vi "FGV FID CH4 Kalibrieren.vi"(10 "Aktionen FID kalibrieren":T1, 11 "Sprachliste":string[][](array[string])) -> (1 "Zustand PMA":string, 2 "Aktionen FID kalibrieren":T1)   [LabVIEW 2020, in "Auto Kalibrieren.lvlib"]
uses:
  Auto Kalibrieren.lvlib
  Aktionen FID kalibrieren.ctl
  Analysator Definition/FGV Analysator Definition Aktionen.ctl
  Aktion FGV CalZustand.ctl
  Seiten/EL3000/FID/Aktion FGV Messwerte_F.ctl
  Aktionen FGV Zustand Kalibrierung.ctl
  Aktionen FGV AutoKAL Daten.ctl
  Seiten/EL3000/Allgemeine VI/FGV Uras26 Aktion.ctl
  Seiten/EL3000/FID/FID Kalibrierung/FID Kalibrieren.ctl
  Seiten/EL3000/Allgemeine VI/Allgemeine VI.lvlib
  Seiten/EL3000/FID/FID.lvlib
  Seiten/EL3000/FID/FID Kalibrierung/FID Kalibrierung.lvlib
  Analysator Definition/Analysator Definition.lvlib
  Seiten/CalGas Aufschaltung/CalGas Aufschaltung.lvlib
  Sprachverwaltung/Sprachverwaltung.lvlib
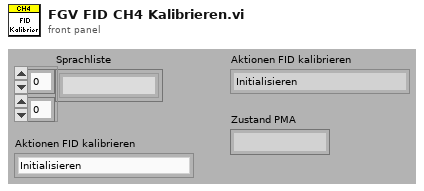
[diagram p1: front panel]
types:
  T1 = typedef "Auto Kalibrieren.lvlib/Aktionen FID kalibrieren.ctl" = enum16{"Initialisieren", "Warten auf FTIR", "Anstehende Störung", "0-Gas Aufschalten", "Nullpunkt Anfordern", "Nullpunkt", "Warten auf andere Messgeräte", "Messgas Aufschalten", "Endpunkt Anfordern", "Endpunkt", "Endpunkt kopieren", "Fertig", "Speichern"}
  T2 = typedef "Analysator Definition.lvlib/FGV Analysator Definition Aktionen.ctl" = enum16{"lesen", "MB setzen", "MB KAL setzen", "laden"}
  T3 = typedef "ABB-EL3000.lvlib/FID.lvlib/Aktion FGV Messwerte_F.ctl" = enum16{"lesen", "Messwerte", "Messbereich", "Status", "Diagnose Werte"}
  T4 = typedef "Auto Kalibrieren.lvlib/Aktion FGV CalZustand.ctl" = enum16{"lesen", "Cal FTIR", "Cal FID CH4", "Cal PMA", "init", "Cal FID THC", "THC CG Eingang"}
  T5 = typedef "Auto Kalibrieren.lvlib/Aktionen FGV Zustand Kalibrierung.ctl" = enum16{"lesen", "LÖSCHEN", "Hintergrund fertig", "Nullpunkt NDIR CO lo", "Endpunkt NDIR CO lo", "Nullpunkt NDIR CO hi", "Endpunkt NDIR CO hi", "Nullpunkt NDIR CO2 lo", "Endpunkt NDIR CO2 lo", "Nullpunkt FID CH4", "Endpunkt FID CH4", "Nullpunkt FID THC", "Endpunkt FID THC", "Nullpunkt PMA", "Endpunkt PMA", "Fehler FT-IR", "Fehler NDIR lo", "Fehler FID CH4", "Fehler FID THC", "Fehler PMA", "TIMEOUT"}
  T6 = typedef "Auto Kalibrieren.lvlib/Aktionen FGV AutoKAL Daten.ctl" = enum16{"lesen", "laden", "speichern", "Aufschaltzeit"}
  T7 = typedef "ABB-EL3000.lvlib/FID.lvlib/FID Kalibrierung.lvlib/FID Kalibrieren.ctl" = enum16{"CH4 Nullpunkt", "THC Nullpunkt", "NMHC Nullpunkt", "CH4 Endpunkt", "THC Endpunkt", "NMHC Endpunkt"}
  T8 = typedef "ABB-EL3000.lvlib/Allgemeine VI.lvlib/FGV Uras26 Aktion.ctl" = enum16{"lesen", "CAL-Daten laden", "Messen", "Kalibrieren vorbereiten", "Kalibrieren", "CAL-Daten speichern", "Toleranz schreiben", "CAL-Daten kopieren"}
  T9 = typedef "Analysator Definition.lvlib/Betriebsdaten Komponente.ctl" = cluster{"Namen":string[], "MB Namen":string[], "Einheit":string, "MB Aktuell":u16, "MB Endwert":u16, "CalGase":u16[], "MB für KAL":u16[], "CG für KAL":u16[]}
  T10 = cluster{"Ausfall":bool, "Funktionskontrolle":bool, "Wartungsbedarf":bool}
  T11 = typedef "Auto Kalibrieren.lvlib/Auschaltzeiten Null Endpunktgase.ctl" = cluster{"CO lo 0":sgl, "CO lo E":sgl, "CO hi 0":sgl, "CO hi E":sgl, "CO2 lo 0":sgl, "CO2 lo E":sgl, "CH4 0":sgl, "CH4 E":sgl, "THC 0":sgl, "THC E":sgl, "O2 0":sgl, "O2 E":sgl}
  T12 = typedef "Auto Kalibrieren.lvlib/Zustand Messgeraete Kalibrierung.ctl" = cluster{"Hintergrund FT-IR":bool, "Nullpunkt NDIR CO lo":bool, "Endpunkt NDIR CO lo":bool, "Nullpunkt NDIR CO hi":bool, "Endpunkt NDIR CO hi":bool, "Nullpunkt NDIR CO2 lo":bool, "Endpunkt NDIR CO2 lo":bool, "Nullpunkt FID CH4":bool, "Endpunkt FID CH4":bool, "Nullpunkt FID THC":bool, "Endpunkt FID THC":bool, "Nullpunkt PMA":bool, "Endpunkt PMA":bool, "Fehler FT-IR":bool, "Fehler NDIR lo":bool, "Fehler FID CH4":bool, "Fehler FID THC":bool, "Fehler PMA":bool}
  T13 = typedef "Zahlen-Ausgabefeld.ctl" = sgl
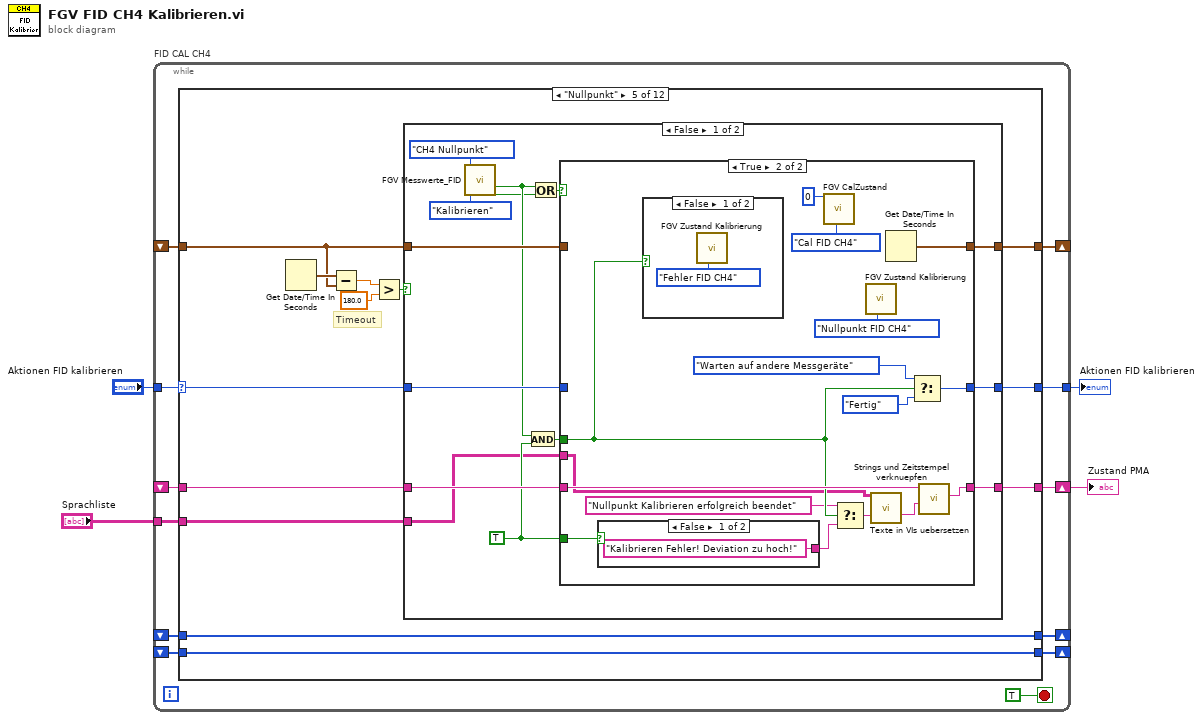
[diagram p0: block diagram]
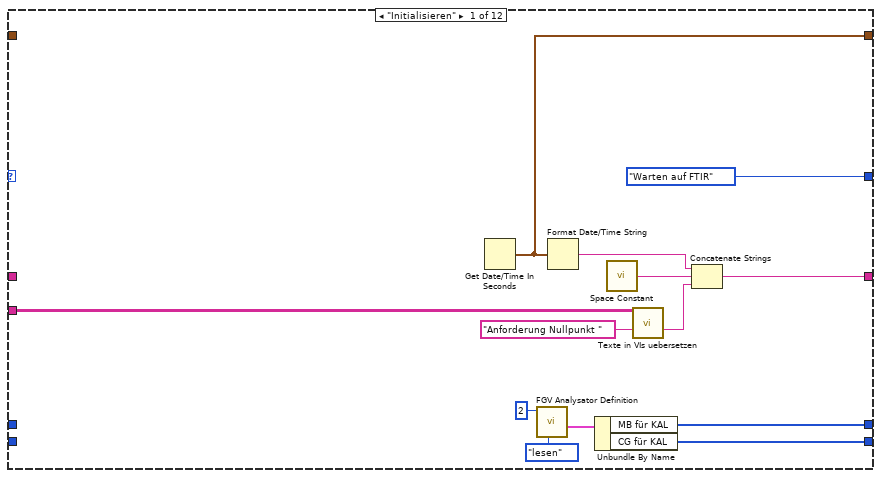
[diagram p2: hidden frame]
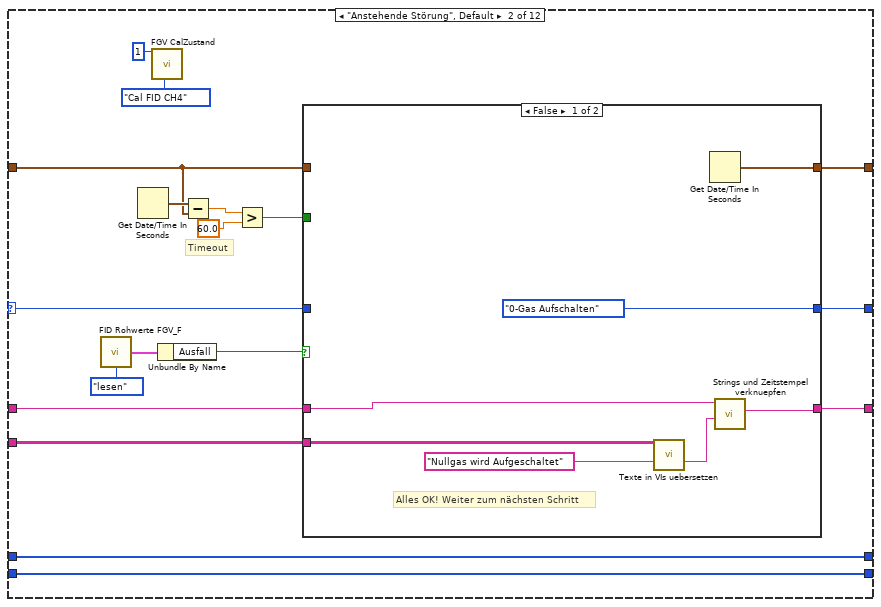
[diagram p3: hidden frame]
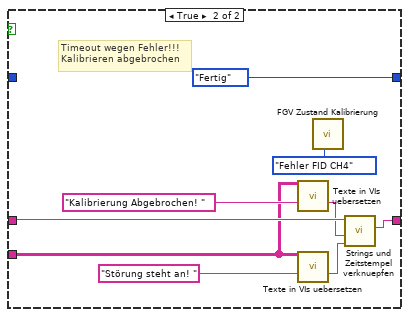
[diagram p5: hidden frame]
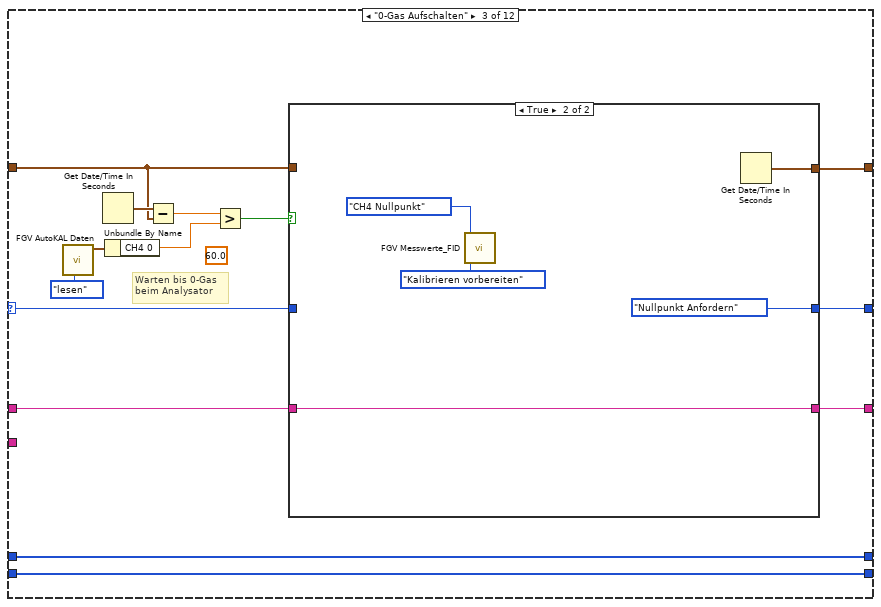
[diagram p6: hidden frame]
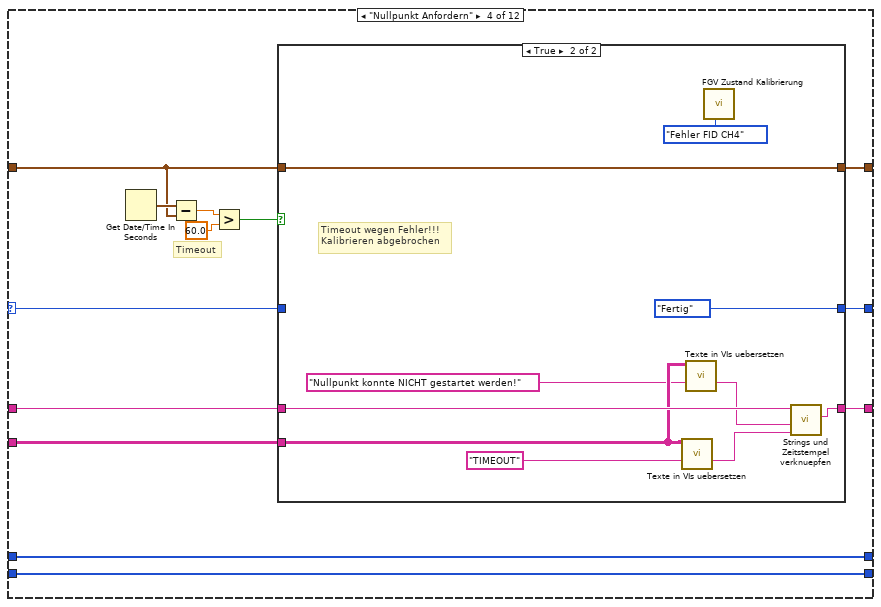
[diagram p8: hidden frame]
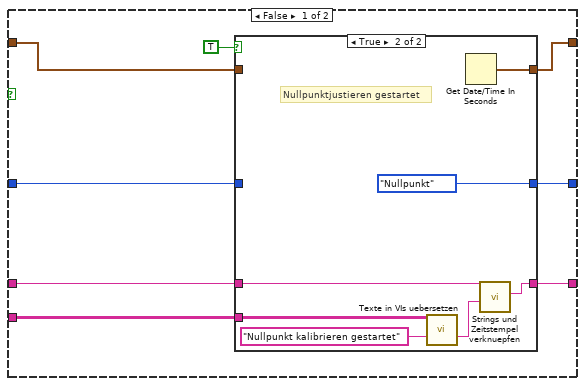
[diagram p9: hidden frame]
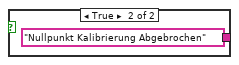
[diagram p12: hidden frame]
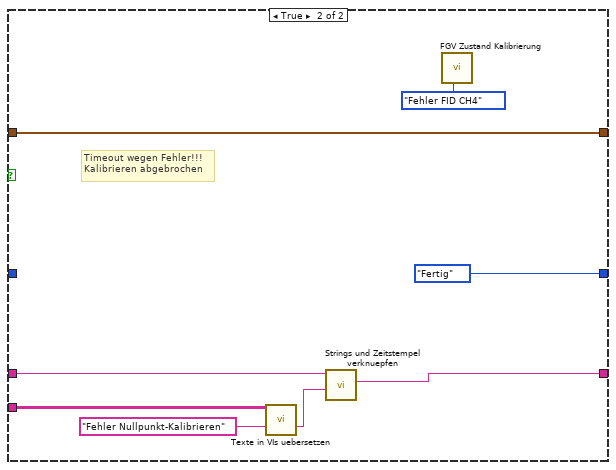
[diagram p14: hidden frame]
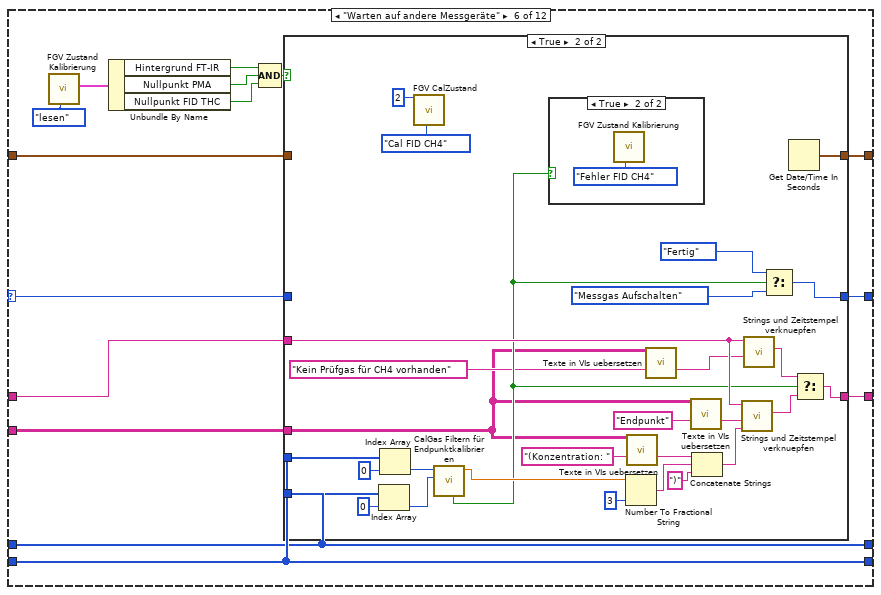
[diagram p15: hidden frame]
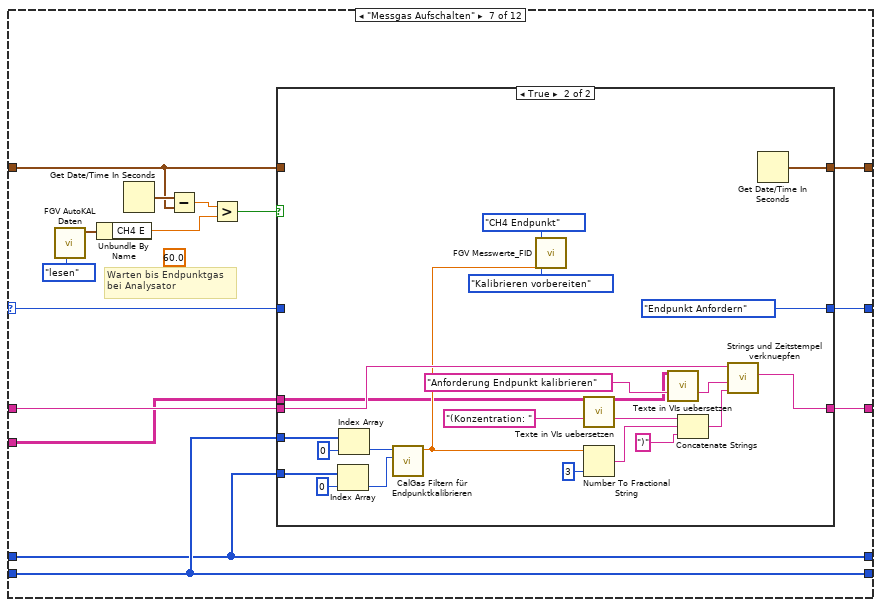
[diagram p18: hidden frame]
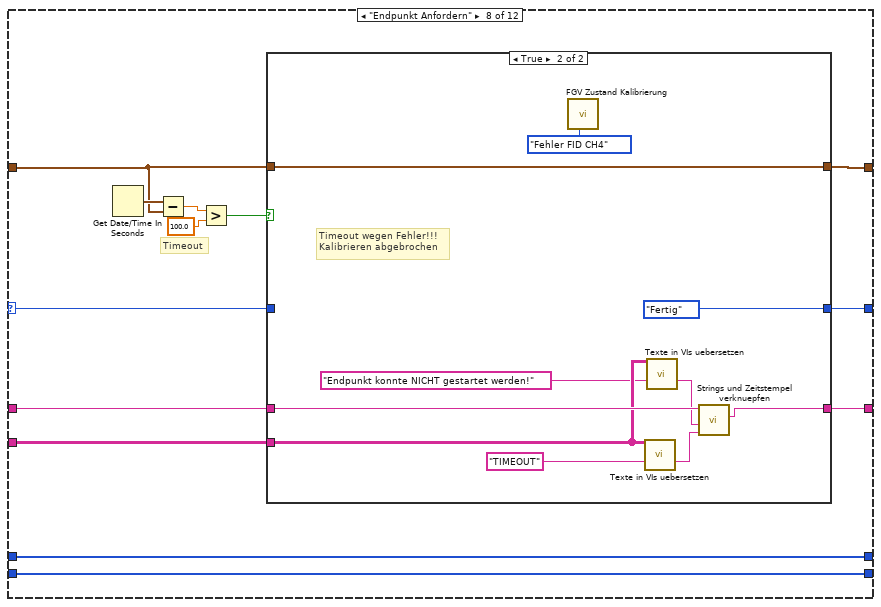
[diagram p20: hidden frame]
diagram:
  n1 = while "FID CAL CH4" {
    shift-right: [w12] -> w4
    shift-left: _ -> [w14]
    shift-right: [w13] -> _
    shift-left: _ -> [w15]
    tunnel: "Aktionen FID kalibrieren" -> [w16]
    tunnel: [w11] -> w2
    shift-right: [w8] -> _
    shift-left: _ -> [w6]
    shift-right: [w9] -> _
    shift-left: _ -> [w7]
    tunnel: "Sprachliste" -> [w5]
    stop <- TRUE stop-if-true
    n2 = case shown="\"Nullpunkt\"" w16 {
      selector: w16 -> [_ w40 w81 w98 w139 w202 w250 w285 w330 w383 _ w404]
      tunnel: w15 -> [_ w38 w83 w103 w141 w203 w253 w290 w332 w384 _ w405]
      tunnel: w14 -> [_ w43 w79 w100 w143 w205 w248 w287 w331 w382 w397 w409]
      tunnel: [w27 w44 w82 w102 w140 w206 w252 w289 w329 w384 w398 w405] -> w13
      tunnel: [w26 w42 w78 w99 w142 w204 w247 w286 w327 w382 w397 w409] -> w12
      tunnel: [Aktionen_FID_kalibrieren."Warten auf FTIR" ("Aktionen FID kalibrieren") w39 w80 w101 w144 w207 w249 w288 w328 w383 Aktionen_FID_kalibrieren."Fertig" ("Aktionen FID kalibrieren") w408] -> w11
      tunnel: [w21 w32 w74 w97 w138 w195 w242 w284 w325 w381 w394 w401] -> w9
      tunnel: [w20 w31 w73 w96 w137 w196 w243 w283 w324 w380 w393 w400] -> w8
      tunnel: w7 -> [_ w32 w74 w97 w138 w195 w242 w284 w325 w381 w394 w401]
      tunnel: w6 -> [_ w31 w73 w96 w137 w196 w243 w283 w324 w380 w393 w400]
      tunnel: w5 -> [w17 w30 _ w95 w136 w193 w241 w282 w323 _ _ _]
      frame "Initialisieren" {
        n3 = Get Date/Time In Seconds() -> (seconds since 1Jan1904=w27:timestamp)
        n4 = call "FGV Analysator Definition.vi"("Aktionen"=FGV_Analysator_Definition_Aktionen."lesen", "Komponente"=2) -> ("Betriebsdaten Komponente"=w23:T9)  [unwired: 5 in, 4 out]
        n5 = Format Date/Time String(seconds (now)=w27) -> (date/time string=w29:string)  [unwired: 2 in]
        n6 = Unbundle By Name(w23) -> ("MB für KAL"=w21:u16[], "CG für KAL"=w20:u16[])
        n7 = call <vilib>:"Space Constant.vi"() -> ("String"=w28:string)
        n8 = call "Texte in VIs uebersetzen.vi"("Sprachliste"=w17, "String zum Übersetzen"="Anforderung Nullpunkt " ("String")) -> ("String zum Übersetzen"=w18:string)  [unwired: 9 in, 4 out]
        n9 = Concatenate Strings(w29, w28, w18) -> (w26:string)
      }
      frame "Anstehende Störung", Default {
        # "Timeout"
        n10 = call "FID Rohwerte FGV_F.vi"("Aktion"=Aktion_FGV_Messwerte_F."lesen") -> ("Status"=w36:T10)  [unwired: 11 in, 3 out]
        n11 = Get Date/Time In Seconds() -> (seconds since 1Jan1904=w47:timestamp)
        n12 = call "FGV CalZustand.vi"("CAL Zustand"=u16 1 ("CAL Zustand FTIR"), "Aktion"=Aktion_FGV_CalZustand."Cal FID CH4") -> ()  [unwired: 13 in, 5 out]
        n13 = Unbundle By Name(w36) -> ("Ausfall"=w37:bool)
        n14 = Subtract(x=w47, y=w38) -> (x-y=w46:dbl)
        n15 = Greater?(x=w46, y=60.0) -> (0:w41:bool)
        n16 = case shown="False" w37 {
          tunnel: [w54 w58] -> w44
          tunnel: w43 -> [w53 w57]
          tunnel: [w52 w56] -> w42
          tunnel: w41 -> [_ w61]
          tunnel: w40 -> [_ w60]
          tunnel: [Aktionen_FID_kalibrieren."0-Gas Aufschalten" ("Aktionen FID kalibrieren") w59] -> w39
          tunnel: w38 -> [_ w58]
          tunnel: w30 -> [w48 w55]
          frame False {
            # "Alles OK! Weiter zum nächsten Schritt"
            n17 = call "Texte in VIs uebersetzen.vi"("Sprachliste"=w48, "String zum Übersetzen"="Nullgas wird Aufgeschaltet" ("String 1 hinzufügen")) -> ("String zum Übersetzen"=w49:string)  [unwired: 9 in, 4 out]
            n18 = Get Date/Time In Seconds() -> (seconds since 1Jan1904=w54:timestamp)
            n19 = call "Strings und Zeitstempel verknuepfen.vi"("String 1 hinzufügen"=w49, "Eingagns String"=w53) -> ("Verknüpfter String"=w52:string)  [unwired: 9 in]
          }
          frame True {
            n20 = case shown="False" w61 {
              tunnel: w60 -> [w63 _]
              tunnel: [w63 Aktionen_FID_kalibrieren."Fertig" ("Aktionen FID kalibrieren")] -> w59
              tunnel: w57 -> [w62 w72]
              tunnel: [w62 w71] -> w56
              tunnel: w55 -> [_ w65]
              frame False {
                # "Fehler steht an!!!!"
              }
              frame True {
                # "Timeout wegen Fehler!!! \nKalibrieren abgebrochen"
                n21 = call "Texte in VIs uebersetzen.vi"("Sprachliste"=w65, "String zum Übersetzen"="Kalibrierung Abgebrochen! " ("String")) -> ("String zum Übersetzen"=w67:string)  [unwired: 9 in, 4 out]
                n22 = call "Texte in VIs uebersetzen.vi"("Sprachliste"=w65, "String zum Übersetzen"="Störung steht an! " ("String")) -> ("String zum Übersetzen"=w66:string)  [unwired: 9 in, 4 out]
                n23 = call "FGV Zustand Kalibrierung.vi"("Aktionen"=Aktionen_FGV_Zustand_Kalibrierung."Fehler FID CH4" ("Enum")) -> ()  [unwired: 9 in, 2 out]
                n24 = call "Strings und Zeitstempel verknuepfen.vi"("String 2 hinzufügen"=w66, "String 1 hinzufügen"=w67, "Eingagns String"=w72) -> ("Verknüpfter String"=w71:string)  [unwired: 8 in]
              }
            }
          }
        }
      }
      frame "0-Gas Aufschalten" {
        (unwired) 60.0 ("y")
        # "Warten bis 0-Gas \nbeim Analysator"
        n25 = call "FGV AutoKAL Daten.vi"("Aktionen"=Aktionen_FGV_AutoKAL_Daten."lesen") -> ("Aufschaltzeiten"=w76:T11)  [unwired: 10 in]
        n26 = Get Date/Time In Seconds() -> (seconds since 1Jan1904=w86:timestamp)
        n27 = Unbundle By Name(w76) -> ("CH4 0"=w75:sgl)
        n28 = Subtract(x=w86, y=w83) -> (x-y=w85:dbl)
        n29 = Greater?(x=w85, y=w75) -> (0:w84:bool)
        n30 = case shown="True" w84 {
          tunnel: w83 -> [w89 _]
          tunnel: [w89 w94] -> w82
          tunnel: w81 -> [w88 _]
          tunnel: [w88 Aktionen_FID_kalibrieren."Nullpunkt Anfordern" ("Aktionen FID kalibrieren")] -> w80
          tunnel: w79 -> [w87 w93]
          tunnel: [w87 w93] -> w78
          frame False {
          }
          frame True {
            n31 = call "FGV Messwerte_FID.vi"("Kalibrieren"=FID_Kalibrieren."CH4 Nullpunkt", "Aktion"=FGV_Uras26_Aktion."Kalibrieren vorbereiten") -> ()  [unwired: 18 in, 8 out]
            n32 = Get Date/Time In Seconds() -> (seconds since 1Jan1904=w94:timestamp)
          }
        }
      }
      frame "Nullpunkt Anfordern" {
        # "Timeout"
        n33 = Get Date/Time In Seconds() -> (seconds since 1Jan1904=w107:timestamp)
        n34 = Subtract(x=w107, y=w103) -> (x-y=w106:dbl)
        n35 = Greater?(x=w106, y=60.0) -> (0:w104:bool)
        n36 = case shown="True" w104 {
          tunnel: w103 -> [w111 w135]
          tunnel: [w110 w135] -> w102
          tunnel: [w113 Aktionen_FID_kalibrieren."Fertig" ("Aktionen FID kalibrieren")] -> w101
          tunnel: w100 -> [w115 w134]
          tunnel: [w114 w133] -> w99
          tunnel: w98 -> [w112 _]
          tunnel: w95 -> [w108 w127]
          frame False {
            n37 = case shown="True" TRUE {
              tunnel: w115 -> [w116 w125]
              tunnel: [w116 w124] -> w114
              tunnel: [w118 Aktionen_FID_kalibrieren."Nullpunkt" ("Aktionen FID kalibrieren")] -> w113
              tunnel: w112 -> [w118 _]
              tunnel: w111 -> [w117 _]
              tunnel: [w117 w123] -> w110
              tunnel: w108 -> [_ w119]
              frame False {
              }
              frame True {
                # "Nullpunktjustieren gestartet"
                n38 = call "Texte in VIs uebersetzen.vi"("Sprachliste"=w119, "String zum Übersetzen"="Nullpunkt kalibrieren gestartet" ("String 1 hinzufügen")) -> ("String zum Übersetzen"=w120:string)  [unwired: 9 in, 4 out]
                n39 = Get Date/Time In Seconds() -> (seconds since 1Jan1904=w123:timestamp)
                n40 = call "Strings und Zeitstempel verknuepfen.vi"("String 1 hinzufügen"=w120, "Eingagns String"=w125) -> ("Verknüpfter String"=w124:string)  [unwired: 9 in]
              }
            }
          }
          frame True {
            # "Timeout wegen Fehler!!! \nKalibrieren abgebrochen"
            n41 = call "Texte in VIs uebersetzen.vi"("Sprachliste"=w127, "String zum Übersetzen"="TIMEOUT" ("String")) -> ("String zum Übersetzen"=w128:string)  [unwired: 9 in, 4 out]
            n42 = call "Texte in VIs uebersetzen.vi"("Sprachliste"=w127, "String zum Übersetzen"="Nullpunkt konnte NICHT gestartet werden!" ("String")) -> ("String zum Übersetzen"=w130:string)  [unwired: 9 in, 4 out]
            n43 = call "FGV Zustand Kalibrierung.vi"("Aktionen"=Aktionen_FGV_Zustand_Kalibrierung."Fehler FID CH4" ("Enum")) -> ()  [unwired: 9 in, 2 out]
            n44 = call "Strings und Zeitstempel verknuepfen.vi"("String 2 hinzufügen"=w128, "String 1 hinzufügen"=w130, "Eingagns String"=w134) -> ("Verknüpfter String"=w133:string)  [unwired: 8 in]
          }
        }
      }
      frame "Nullpunkt" {
        # "Timeout"
        n45 = Get Date/Time In Seconds() -> (seconds since 1Jan1904=w148:timestamp)
        n46 = Subtract(x=w148, y=w141) -> (x-y=w147:dbl)
        n47 = Greater?(x=w147, y=180.0) -> (0:w145:bool)
        n48 = case shown="False" w145 {
          tunnel: [w159 Aktionen_FID_kalibrieren."Fertig" ("Aktionen FID kalibrieren")] -> w144
          tunnel: w143 -> [w158 w192]
          tunnel: [w157 w191] -> w142
          tunnel: w141 -> [w162 w190]
          tunnel: [w161 w190] -> w140
          tunnel: w139 -> [w160 _]
          tunnel: w136 -> [w149 w186]
          frame False {
            w154 = TRUE
            n49 = call "FGV Messwerte_FID.vi"("Kalibrieren"=FID_Kalibrieren."CH4 Nullpunkt", "Aktion"=FGV_Uras26_Aktion."Kalibrieren") -> ("Kalibrieren erfolgreich"=w151:bool, "CAL TimeOut"=w150:bool)  [unwired: 18 in, 6 out]
            n50 = And(x=w151, y=w154) -> (x .and. y?=w155:bool)
            n51 = Or(x=w151, y=w150) -> (x .or. y?=w156:bool)
            n52 = case shown="True" w156 {
              tunnel: w162 -> [w165 _]
              tunnel: [w165 w177] -> w161
              tunnel: w160 -> [w164 _]
              tunnel: [w164 w178] -> w159
              tunnel: w158 -> [w163 w181]
              tunnel: [w163 w180] -> w157
              tunnel: w155 -> [_ w175]
              tunnel: w154 -> [_ w174]
              tunnel: w149 -> [_ w167]
              frame False {
              }
              frame True {
                n53 = case shown="False" w174 {
                  tunnel: ["Kalibrieren Fehler! Deviation zu hoch!" ("String 1 hinzufügen") "Nullpunkt Kalibrierung Abgebrochen" ("String 1 hinzufügen")] -> w179
                  frame False {
                  }
                  frame True {
                  }
                }
                n54 = case shown="False" w175 {
                  frame False {
                    n55 = call "FGV Zustand Kalibrierung.vi"("Aktionen"=Aktionen_FGV_Zustand_Kalibrierung."Fehler FID CH4" ("Enum")) -> ()  [unwired: 9 in, 2 out]
                  }
                  frame True {
                  }
                }
                n56 = call "FGV CalZustand.vi"("CAL Zustand"=u16 0 ("CAL Zustand FTIR"), "Aktion"=Aktion_FGV_CalZustand."Cal FID CH4") -> ()  [unwired: 13 in, 5 out]
                n57 = Select(t="Nullpunkt Kalibrieren erfolgreich beendet" ("String 1 hinzufügen"), s=w175, f=w179) -> (s? t:f=w169:string)
                n58 = call "FGV Zustand Kalibrierung.vi"("Aktionen"=Aktionen_FGV_Zustand_Kalibrierung."Nullpunkt FID CH4" ("Enum")) -> ()  [unwired: 9 in, 2 out]
                n59 = call "Texte in VIs uebersetzen.vi"("Sprachliste"=w167, "String zum Übersetzen"=w169) -> ("String zum Übersetzen"=w168:string)  [unwired: 9 in, 4 out]
                n60 = Get Date/Time In Seconds() -> (seconds since 1Jan1904=w177:timestamp)
                n61 = Select(t=Aktionen_FID_kalibrieren."Warten auf andere Messgeräte" ("Aktionen FID kalibrieren"), s=w175, f=Aktionen_FID_kalibrieren."Fertig" ("Aktionen FID kalibrieren")) -> (s? t:f=w178:T1)
                n62 = call "Strings und Zeitstempel verknuepfen.vi"("String 1 hinzufügen"=w168, "Eingagns String"=w181) -> ("Verknüpfter String"=w180:string)  [unwired: 9 in]
              }
            }
          }
          frame True {
            # "Timeout wegen Fehler!!! \nKalibrieren abgebrochen"
            n63 = call "Texte in VIs uebersetzen.vi"("Sprachliste"=w186, "String zum Übersetzen"="Fehler Nullpunkt-Kalibrieren" ("String 1 hinzufügen")) -> ("String zum Übersetzen"=w187:string)  [unwired: 9 in, 4 out]
            n64 = call "Strings und Zeitstempel verknuepfen.vi"("String 1 hinzufügen"=w187, "Eingagns String"=w192) -> ("Verknüpfter String"=w191:string)  [unwired: 9 in]
            n65 = call "FGV Zustand Kalibrierung.vi"("Aktionen"=Aktionen_FGV_Zustand_Kalibrierung."Fehler FID CH4" ("Enum")) -> ()  [unwired: 9 in, 2 out]
          }
        }
      }
      frame "Warten auf andere Messgeräte" {
        n66 = call "FGV Zustand Kalibrierung.vi"("Aktionen"=Aktionen_FGV_Zustand_Kalibrierung."lesen" ("Enum")) -> ("Zustand Kalibrierung"=w200:T12)  [unwired: 9 in, 1 out]
        n67 = Unbundle By Name(w200) -> ("Hintergrund FT-IR"=w199:bool, "Nullpunkt PMA"=w197:bool, "Nullpunkt FID THC"=w194:bool)
        n68 = Compound Arithmetic op=AND(w199, w197, w194) -> (w198:bool)
        n69 = case shown="True" w198 {
          tunnel: [w209 w234] -> w207
          tunnel: [w210 w239] -> w206
          tunnel: w205 -> [w208 w236]
          tunnel: [w208 w235] -> w204
          tunnel: w203 -> [w210 _]
          tunnel: w202 -> [w209 _]
          tunnel: w196 -> [_ w219]
          tunnel: w195 -> [_ w218]
          tunnel: w193 -> [_ w211]
          frame False {
          }
          frame True {
            n70 = Index Array(array=w218, index=0 ("Index")) -> (element=w222:u16)
            n71 = Index Array(array=w219, index=0 ("Index")) -> (element=w223:u16)
            n72 = call "FGV CalZustand.vi"("CAL Zustand"=u16 2 ("CAL Zustand FTIR"), "Aktion"=Aktion_FGV_CalZustand."Cal FID CH4") -> ()  [unwired: 13 in, 5 out]
            n73 = call "CalGas Filtern für Endpunktkalibrieren.vi"("Messbereich"=w222, "CalGas"=w223) -> ("Wert 1"=w221:T13, "Fehler"=w220:bool)  [unwired: 2 in, 6 out]
            n74 = case shown="True" w220 {
              frame False {
              }
              frame True {
                n75 = call "FGV Zustand Kalibrierung.vi"("Aktionen"=Aktionen_FGV_Zustand_Kalibrierung."Fehler FID CH4" ("Enum")) -> ()  [unwired: 9 in, 2 out]
              }
            }
            n76 = Number To Fractional String(number=w221, precision (6)=i16 3 ("Genauigkeit (6)")) -> (F-format string=w232:string)  [unwired: 2 in]
            n77 = call "Texte in VIs uebersetzen.vi"("Sprachliste"=w211, "String zum Übersetzen"="(Konzentration: " ("String")) -> ("String zum Übersetzen"=w212:string)  [unwired: 9 in, 4 out]
            n78 = call "Texte in VIs uebersetzen.vi"("Sprachliste"=w211, "String zum Übersetzen"="Kein Prüfgas für CH4 vorhanden" ("String 1 hinzufügen")) -> ("String zum Übersetzen"=w216:string)  [unwired: 9 in, 4 out]
            n79 = call "Texte in VIs uebersetzen.vi"("Sprachliste"=w211, "String zum Übersetzen"="Endpunkt" ("String 1 hinzufügen")) -> ("String zum Übersetzen"=w214:string)  [unwired: 9 in, 4 out]
            n80 = Concatenate Strings(w212, w232, ")" ("String")) -> (w237:string)
            n81 = call "Strings und Zeitstempel verknuepfen.vi"("String 2 hinzufügen"=w237, "String 1 hinzufügen"=w214, "Eingagns String"=w236) -> ("Verknüpfter String"=w230:string)  [unwired: 8 in]
            n82 = call "Strings und Zeitstempel verknuepfen.vi"("String 1 hinzufügen"=w216, "Eingagns String"=w236) -> ("Verknüpfter String"=w231:string)  [unwired: 9 in]
            n83 = Select(t=Aktionen_FID_kalibrieren."Fertig" ("Aktionen FID kalibrieren"), s=w220, f=Aktionen_FID_kalibrieren."Messgas Aufschalten" ("Aktionen FID kalibrieren")) -> (s? t:f=w234:T1)
            n84 = Get Date/Time In Seconds() -> (seconds since 1Jan1904=w239:timestamp)
            n85 = Select(t=w231, s=w220, f=w230) -> (s? t:f=w235:string)
          }
        }
      }
      frame "Messgas Aufschalten" {
        (unwired) 60.0 ("y")
        # "Warten bis Endpunktgas\nbei Analysator"
        n86 = call "FGV AutoKAL Daten.vi"("Aktionen"=Aktionen_FGV_AutoKAL_Daten."lesen") -> ("Aufschaltzeiten"=w245:T11)  [unwired: 10 in]
        n87 = Unbundle By Name(w245) -> ("CH4 E"=w244:sgl)
        n88 = Get Date/Time In Seconds() -> (seconds since 1Jan1904=w255:timestamp)
        n89 = Subtract(x=w255, y=w253) -> (x-y=w254:dbl)
        n90 = Greater?(x=w254, y=w244) -> (0:w251:bool)
        n91 = case shown="True" w251 {
          tunnel: w253 -> [w258 _]
          tunnel: [w258 w277] -> w252
          tunnel: w250 -> [w257 _]
          tunnel: [w257 Aktionen_FID_kalibrieren."Endpunkt Anfordern" ("Aktionen FID kalibrieren")] -> w249
          tunnel: w248 -> [w256 w278]
          tunnel: [w256 w279] -> w247
          tunnel: w243 -> [_ w269]
          tunnel: w242 -> [_ w268]
          tunnel: w241 -> [_ w260]
          frame False {
          }
          frame True {
            n92 = Index Array(array=w268, index=0 ("Index")) -> (element=w270:u16)
            n93 = Index Array(array=w269, index=0 ("Index")) -> (element=w271:u16)
            n94 = call "CalGas Filtern für Endpunktkalibrieren.vi"("Messbereich"=w270, "CalGas"=w271) -> ("Wert 1"=w265:T13)  [unwired: 2 in, 7 out]
            n95 = call "FGV Messwerte_FID.vi"("Prüfgaskonz."=w265, "Kalibrieren"=FID_Kalibrieren."CH4 Endpunkt", "Aktion"=FGV_Uras26_Aktion."Kalibrieren vorbereiten") -> ()  [unwired: 17 in, 8 out]
            n96 = call "Texte in VIs uebersetzen.vi"("Sprachliste"=w260, "String zum Übersetzen"="(Konzentration: " ("String")) -> ("Sprachliste out"=w259:string[][], "String zum Übersetzen"=w261:string)  [unwired: 9 in, 3 out]
            n97 = Number To Fractional String(number=w265, precision (6)=i16 3 ("Genauigkeit (6)")) -> (F-format string=w275:string)  [unwired: 2 in]
            n98 = call "Texte in VIs uebersetzen.vi"("Sprachliste"=w259, "String zum Übersetzen"="Anforderung Endpunkt kalibrieren" ("String 1 hinzufügen")) -> ("String zum Übersetzen"=w263:string)  [unwired: 9 in, 4 out]
            n99 = Concatenate Strings(w261, w275, ")" ("String")) -> (w280:string)
            n100 = call "Strings und Zeitstempel verknuepfen.vi"("String 2 hinzufügen"=w280, "String 1 hinzufügen"=w263, "Eingagns String"=w278) -> ("Verknüpfter String"=w279:string)  [unwired: 8 in]
            n101 = Get Date/Time In Seconds() -> (seconds since 1Jan1904=w277:timestamp)
          }
        }
      }
      frame "Endpunkt Anfordern" {
        # "Timeout"
        n102 = Get Date/Time In Seconds() -> (seconds since 1Jan1904=w294:timestamp)
        n103 = Subtract(x=w294, y=w290) -> (x-y=w293:dbl)
        n104 = Greater?(x=w293, y=100.0) -> (0:w291:bool)
        n105 = case shown="True" w291 {
          tunnel: w290 -> [w302 w322]
          tunnel: [w297 w322] -> w289
          tunnel: [w298 Aktionen_FID_kalibrieren."Fertig" ("Aktionen FID kalibrieren")] -> w288
          tunnel: w287 -> [w300 w321]
          tunnel: [w299 w320] -> w286
          tunnel: w285 -> [w301 _]
          tunnel: w282 -> [w295 w314]
          frame False {
            n106 = case shown="True" TRUE {
              tunnel: w300 -> [w303 w312]
              tunnel: [w303 w311] -> w299
              tunnel: [w305 Aktionen_FID_kalibrieren."Endpunkt" ("Aktionen FID kalibrieren")] -> w298
              tunnel: w301 -> [w305 _]
              tunnel: w302 -> [w304 _]
              tunnel: [w304 w310] -> w297
              tunnel: w295 -> [_ w306]
              frame False {
              }
              frame True {
                # "Endpunkt Kalibrieren gestartet"
                n107 = call "Texte in VIs uebersetzen.vi"("Sprachliste"=w306, "String zum Übersetzen"="Endpunkt kalibrieren gestartet" ("String 1 hinzufügen")) -> ("String zum Übersetzen"=w307:string)  [unwired: 9 in, 4 out]
                n108 = call "Strings und Zeitstempel verknuepfen.vi"("String 1 hinzufügen"=w307, "Eingagns String"=w312) -> ("Verknüpfter String"=w311:string)  [unwired: 9 in]
                n109 = Get Date/Time In Seconds() -> (seconds since 1Jan1904=w310:timestamp)
              }
            }
          }
          frame True {
            # "Timeout wegen Fehler!!! \nKalibrieren abgebrochen"
            n110 = call "FGV Zustand Kalibrierung.vi"("Aktionen"=Aktionen_FGV_Zustand_Kalibrierung."Fehler FID CH4" ("Enum")) -> ()  [unwired: 9 in, 2 out]
            n111 = call "Texte in VIs uebersetzen.vi"("Sprachliste"=w314, "String zum Übersetzen"="TIMEOUT" ("String")) -> ("String zum Übersetzen"=w315:string)  [unwired: 9 in, 4 out]
            n112 = call "Texte in VIs uebersetzen.vi"("Sprachliste"=w314, "String zum Übersetzen"="Endpunkt konnte NICHT gestartet werden!" ("String")) -> ("String zum Übersetzen"=w317:string)  [unwired: 9 in, 4 out]
            n113 = call "Strings und Zeitstempel verknuepfen.vi"("String 2 hinzufügen"=w315, "String 1 hinzufügen"=w317, "Eingagns String"=w321) -> ("Verknüpfter String"=w320:string)  [unwired: 8 in]
          }
        }
      }
      frame "Endpunkt" {
        # "Timeout"
        n114 = Get Date/Time In Seconds() -> (seconds since 1Jan1904=w335:timestamp)
        n115 = Subtract(x=w335, y=w332) -> (x-y=w334:dbl)
        n116 = Greater?(x=w334, y=180.0) -> (0:w326:bool)
        n117 = case shown="False" w326 {
          tunnel: [w346 Aktionen_FID_kalibrieren."Fertig" ("Aktionen FID kalibrieren")] -> w328
          tunnel: w331 -> [w345 w377]
          tunnel: [w344 w376] -> w327
          tunnel: w332 -> [w349 w375]
          tunnel: [w348 w375] -> w329
          tunnel: w330 -> [w347 _]
          tunnel: w323 -> [w336 w370]
          frame False {
            w341 = TRUE
            n118 = call "FGV Messwerte_FID.vi"("Kalibrieren"=FID_Kalibrieren."CH4 Endpunkt", "Aktion"=FGV_Uras26_Aktion."Kalibrieren") -> ("Kalibrieren erfolgreich"=w338:bool, "CAL TimeOut"=w337:bool)  [unwired: 18 in, 6 out]
            n119 = Or(x=w338, y=w337) -> (x .or. y?=w343:bool)
            n120 = And(x=w338, y=w341) -> (x .and. y?=w342:bool)
            n121 = case shown="True" w343 {
              tunnel: w349 -> [w352 _]
              tunnel: [w352 w363] -> w348
              tunnel: w347 -> [w351 _]
              tunnel: [w351 w361] -> w346
              tunnel: w345 -> [w350 w366]
              tunnel: [w350 w365] -> w344
              tunnel: w342 -> [_ w360]
              tunnel: w341 -> [_ w359]
              tunnel: w336 -> [_ w354]
              frame False {
              }
              frame True {
                n122 = case shown="True" w359 {
                  tunnel: ["Kalibriern Fehler! Deviation zu Hoch!" ("String 1 hinzufügen") "Endpunkt Kalibrierung abgebrochen!" ("String 1 hinzufügen")] -> w364
                  frame False {
                  }
                  frame True {
                  }
                }
                n123 = case shown="False" w360 {
                  frame False {
                    n124 = call "FGV Zustand Kalibrierung.vi"("Aktionen"=Aktionen_FGV_Zustand_Kalibrierung."Fehler FID CH4" ("Enum")) -> ()  [unwired: 9 in, 2 out]
                  }
                  frame True {
                  }
                }
                n125 = Select(t="Endpunkt Kalibrierung erfolgreich beendet" ("String 1 hinzufügen"), s=w360, f=w364) -> (s? t:f=w356:string)
                n126 = Get Date/Time In Seconds() -> (seconds since 1Jan1904=w363:timestamp)
                n127 = call "Texte in VIs uebersetzen.vi"("Sprachliste"=w354, "String zum Übersetzen"=w356) -> ("String zum Übersetzen"=w355:string)  [unwired: 9 in, 4 out]
                n128 = call "FGV Zustand Kalibrierung.vi"("Aktionen"=Aktionen_FGV_Zustand_Kalibrierung."Endpunkt FID CH4" ("Enum")) -> ()  [unwired: 9 in, 2 out]
                n129 = Select(t=Aktionen_FID_kalibrieren."Fertig" ("Aktionen FID kalibrieren"), s=w360, f=Aktionen_FID_kalibrieren."Speichern" ("Aktionen FID kalibrieren")) -> (s? t:f=w361:T1)
                n130 = call "Strings und Zeitstempel verknuepfen.vi"("String 1 hinzufügen"=w355, "Eingagns String"=w366) -> ("Verknüpfter String"=w365:string)  [unwired: 9 in]
              }
            }
          }
          frame True {
            # "Timeout wegen Fehler!!! \nKalibrieren abgebrochen"
            n131 = call "FGV Zustand Kalibrierung.vi"("Aktionen"=Aktionen_FGV_Zustand_Kalibrierung."Fehler FID CH4" ("Enum")) -> ()  [unwired: 9 in, 2 out]
            n132 = call "Texte in VIs uebersetzen.vi"("Sprachliste"=w370, "String zum Übersetzen"="Fehler Endpunkt-Kalibrieren" ("String 1 hinzufügen")) -> ("String zum Übersetzen"=w371:string)  [unwired: 9 in, 4 out]
            n133 = call "Strings und Zeitstempel verknuepfen.vi"("String 1 hinzufügen"=w371, "Eingagns String"=w377) -> ("Verknüpfter String"=w376:string)  [unwired: 9 in]
          }
        }
      }
      frame "Fertig" {
        n134 = disable-structure shown="Aktiviert" {
          frame Disabled {
            n135 = call "FGV Zustand Kalibrierung.vi"("Aktionen"=Aktionen_FGV_Zustand_Kalibrierung."lesen" ("Enum")) -> ("Zustand Kalibrierung"=w388:T12)  [unwired: 9 in, 1 out]
            n136 = Unbundle By Name(w388) -> ("Nullpunkt FID CH4"=w387:bool, "Endpunkt FID CH4"=w386:bool)
            n137 = And(x=w387, y=w386) -> (x .and. y?=w385:bool)
            n138 = case shown="True" w385 {
              frame False {
              }
              frame True {
                n139 = call "FGV CalZustand.vi"("CAL Zustand"=u16 0 ("CAL Zustand FTIR"), "Aktion"=Aktion_FGV_CalZustand."Cal FID CH4") -> ()  [unwired: 13 in, 5 out]
              }
            }
          }
          frame Enabled {
          }
        }
        n140 = call "FGV CalZustand.vi"("CAL Zustand"=u16 0 ("CAL Zustand FTIR"), "Aktion"=Aktion_FGV_CalZustand."Cal FID CH4") -> ()  [unwired: 13 in, 5 out]
      }
      frame "Speichern" {
        n141 = call "FGV Zustand Kalibrierung.vi"("Aktionen"=Aktionen_FGV_Zustand_Kalibrierung."Endpunkt FID CH4" ("Enum")) -> ()  [unwired: 9 in, 2 out]
        n142 = call "FGV Messwerte_FID.vi"("Aktion"=FGV_Uras26_Aktion."CAL-Daten speichern") -> ()  [unwired: 19 in, 8 out]
        n143 = Get Date/Time In Seconds() -> (seconds since 1Jan1904=w398:timestamp)
      }
      frame "Warten auf FTIR" {
        n144 = call "FGV Zustand Kalibrierung.vi"("Aktionen"=Aktionen_FGV_Zustand_Kalibrierung."lesen" ("Enum")) -> ("Zustand Kalibrierung"=w406:T12)  [unwired: 9 in, 1 out]
        n145 = Unbundle By Name(w406) -> ()  [unwired: 1 out]
        n146 = call "FGV CalZustand.vi"("CAL Zustand"=u16 1 ("CAL Zustand FTIR"), "Aktion"=Aktion_FGV_CalZustand."Cal FID CH4") -> ()  [unwired: 13 in, 5 out]
        n147 = case shown="True" TRUE {
          tunnel: [w410 Aktionen_FID_kalibrieren."Anstehende Störung" ("Aktionen FID kalibrieren")] -> w408
          tunnel: w404 -> [w410 _]
          frame False {
          }
          frame True {
          }
        }
      }
    }
  }
  "Zustand PMA" <- w4
  "Aktionen FID kalibrieren" <- w2
